vi "Enqueue system notification.vi"(8 "error in (no error)":errorcluster, 10 "Message Data":variant, 11 "system message":string) -> (0 "error out":errorcluster)   [LabVIEW 2016, in "Message Queue.lvlib"]
uses:
  Message Queue.lvlib
  System notification queue name (constant).ctl
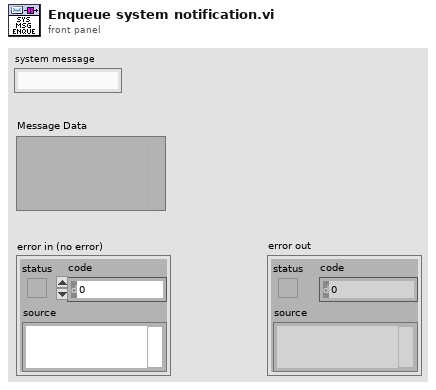
[diagram p1: front panel]
types:
  T1 = typedef "Message Queue.lvlib/System notification queue name (constant).ctl" = string
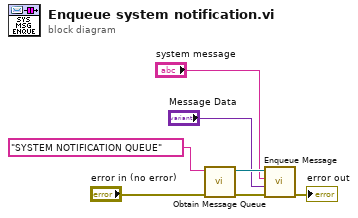
[diagram p0: block diagram]
diagram:
  n1 = call "Obtain Message Queue.vi"("error in (no error)"="error in (no error)", "name (unnamed)"=T1 "SYSTEM NOTIFICATION QUEUE") -> ("error out"=w4:errorcluster, "Message Queue"=w6:refnum<queue>)  [unwired: 7 in, 1 out]
  n2 = call "Enqueue Message.vi"("error in (no error)"=w4, "Message Data"="Message Data", "Message"="system message", "Message Queue"=w6) -> ("error out"=→"error out":errorcluster)  [unwired: 6 in, 1 out]
